vi "Interpolate Quaternions.vi"(1 "ratio":dbl, 2 "quaternion 2":T1, 3 "quaternion 1":T1) -> (0 "interpolated quaternion":T1)   [LabVIEW 2017, in "NI_Kinematics.lvlib"]
doc: "Returns a quaternion that is a spherical linear interpolation between two quaternions.\n\n<B>.m file:</B> qinterp"
uses:
  <vilib>/robotics/Kinematics/NI_Kinematics.lvlib
  <vilib>/robotics/Kinematics/Quaternion.ctl
  <vilib>/Analysis/baseanly.llb/Real Dot Product.vi
  <vilib>/Analysis/NI_AALBase.lvlib
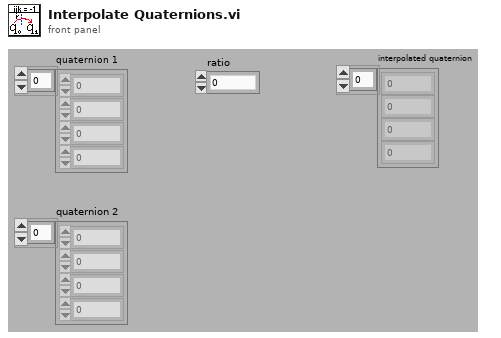
[diagram p1: front panel]
types:
  T1 = typedef "NI_Kinematics.lvlib/Quaternion.ctl" = dbl[]
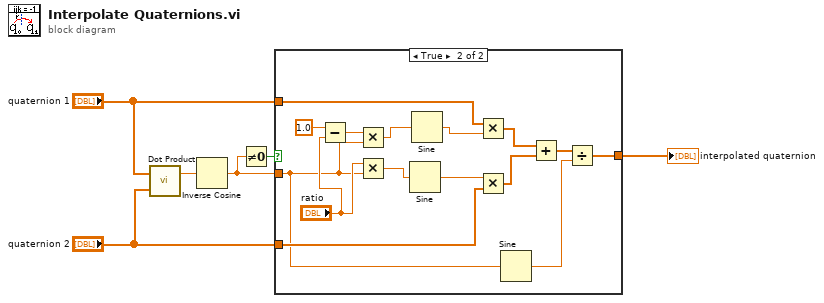
[diagram p0: block diagram]
diagram:
  n1 = call-poly <vilib>:"Dot Product.vi"("Y Vector"="quaternion 2", "X Vector"="quaternion 1") -> ("X * Y"=w6:dbl)  [unwired: 1 out]
  n2 = Inverse Cosine(1:w6) -> (0:w1:dbl)
  n3 = Not Equal To 0?(x=w1) -> (x != 0?=w2:bool)
  n4 = case shown="True" w2 {
    tunnel: "quaternion 1" -> [w7 w22]
    tunnel: "quaternion 2" -> [_ w21]
    tunnel: w1 -> [_ w9]
    tunnel: [w7 w10] -> w3
    frame False {
      # "q1 = q2"
    }
    frame True {
      n5 = Subtract(x=1.0, y="ratio") -> (x-y=w20:dbl)
      n6 = Multiply(x=w20, y=w9) -> (x*y=w17:dbl)
      n7 = Multiply(x="ratio", y=w9) -> (x*y=w14:dbl)
      n8 = Sine(x=w14) -> (sin(x)=w15:dbl)
      n9 = Sine(x=w17) -> (sin(x)=w16:dbl)
      n10 = Multiply(x=w22, y=w16) -> (x*y=w13:T1)
      n11 = Multiply(x=w15, y=w21) -> (x*y=w12:T1)
      n12 = Sine(x=w9) -> (sin(x)=w8:dbl)
      n13 = Add(x=w13, y=w12) -> (x+y=w11:T1)
      n14 = Divide(x=w11, y=w8) -> (x/y=w10:T1)
    }
  }
  "interpolated quaternion" <- w3
